vi "Handle Exception.vi"(7 "Processing In":refnum<class "Processing.lvclass">, 8 "error in (no error)":errorcluster, 11 "Authentication Handler in":refnum<class "Authentication Handler.lvclass">) -> (0 "error out":errorcluster, 5 "Processing":refnum<class "Processing.lvclass">)   [LabVIEW 2020, in "HTTP Server.lvlib" / "Authentication Handler.lvclass"]
uses:
  Authentication Handler.lvclass
  Processing/Processing.lvclass
  User/User.lvclass
  C:/dev/lv20CE/relink/lv-http-server/HTTP Server/Service/Service.lvclass
  Processing/Processing.lvclass/Processing.ctl
  Authentication Provider/Authentication Provider.lvclass
  lv-http-util/HTTP Utils/Redirect Response/Redirect Response.lvclass
  C:/dev/lv20CE/relink/lv-http-util/HTTP Utils/Response/Response.lvclass
  Authentication Handler.lvclass/Authentication Handler.ctl
  lv-http-util/HTTP Utils/Response/Response.lvclass
  lv-http-util/HTTP Utils/Request/Request.lvclass
  Session/Session.lvclass
  Values/Values.lvclass
  lv-uri/URI/URI/URI.lvclass
  C:/dev/lv20CE/relink/lv-http-server/HTTP Server/User/User.lvclass
  C:/dev/lv20CE/relink/lv-http-server/HTTP Server/Authentication Provider/Authentication Provider.lvclass
  C:/dev/lv20CE/relink/lv-http-util/HTTP Utils/Redirect Response/Redirect Response.lvclass
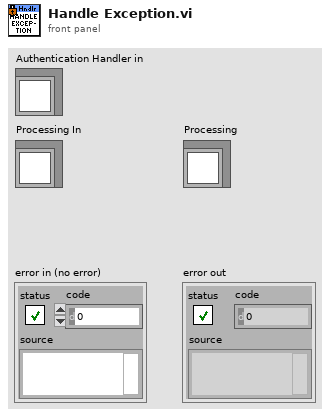
[diagram p1: front panel]
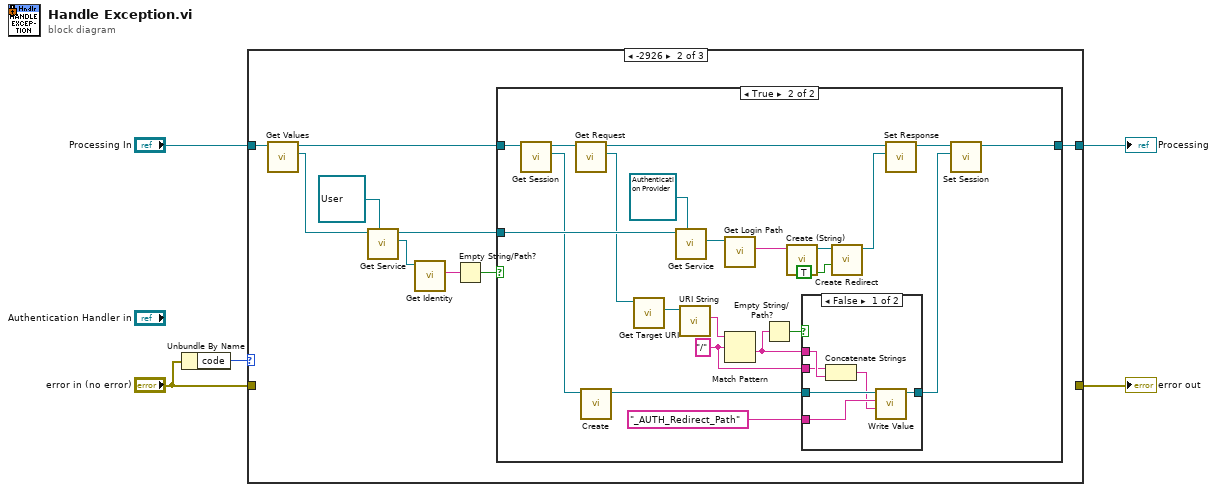
[diagram p0: block diagram]
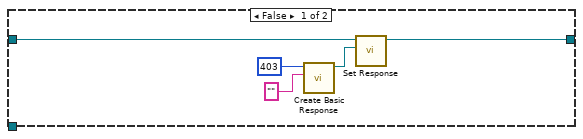
[diagram p3: hidden frame]
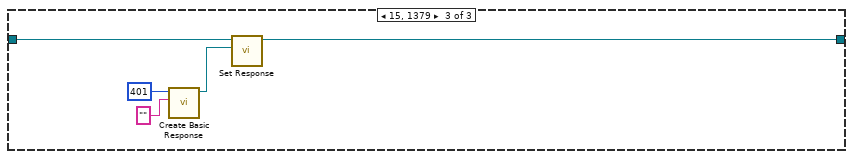
[diagram p5: hidden frame]
diagram:
  n1 = Unbundle By Name("error in (no error)") -> ("code"=w5:i32)
  n2 = case shown="-2926" w5 {
    tunnel: "error in (no error)" -> [w7 _ _]
    tunnel: [w7 _ _] -> w3
    tunnel: "Processing In" -> [w6 w10 w53]
    tunnel: [w6 w11 w51] -> w1
    frame Default {
    }
    frame -2926 {
      n3 = call "Get Values.vi"("Processing in"=w10) -> ("Values"=w9:refnum<class "Values.lvclass">, "Processing out"=w8:refnum<class "Processing.lvclass">)  [unwired: 9 in]
      n4 = call "Get Service.vi"("Service Type"=refnum<class "User.lvclass"> refnum ("HTTP Server.lvlib:User.lvclass"), "Values in"=w9) -> ("Service"=w15:refnum<class "User.lvclass">, "Values out"=w12:refnum<class "Values.lvclass">)  [unwired: 7 in, 1 out]
      n5 = call-dynamic "Get Identity.vi"("User in"=w15) -> ("Identity"=w14:string)  [unwired: 8 in, 2 out]
      n6 = Empty String/Path?(string/path=w14) -> (empty?=w13:bool)
      n7 = case shown="True" w13 {
        tunnel: w12 -> [_ w43]
        tunnel: [w18 w29] -> w11
        tunnel: w8 -> [w17 w25]
        frame False {
          n8 = call "Create Basic Response.vi"("Payload"="", "Status Code"=u16 403) -> ("Response out"=w19:refnum<class "Response.lvclass">)  [unwired: 8 in, 1 out]
          n9 = call "Set Response.vi"("Response"=w19, "Processing in"=w17) -> ("Processing out"=w18:refnum<class "Processing.lvclass">)  [unwired: 9 in]
        }
        frame True {
          w34 = "/" ("regular expression")
          n10 = call "Get Session.vi"("Processing in"=w25) -> ("Session"=w26:refnum<class "Session.lvclass">, "Processing out"=w27:refnum<class "Processing.lvclass">)  [unwired: 9 in]
          n11 = call "Get Request.vi"("Processing in"=w27) -> ("Request"=w33:refnum<class "Request.lvclass">, "Processing out"=w32:refnum<class "Processing.lvclass">)  [unwired: 9 in]
          n12 = call "Create.vi"("Session in"=w26) -> ("Session out"=w28:refnum<class "Session.lvclass">)  [unwired: 9 in, 1 out]
          n13 = call "Get Target URI.vi"("Request in"=w33) -> ("Target URI"=w39:refnum<class "URI.lvclass">)  [unwired: 8 in, 2 out]
          n14 = call "Get Service.vi"("Service Type"=refnum<class "Authentication Provider.lvclass"> refnum ("HTTP Server.lvlib:Authentication Provider.lvclass"), "Values in"=w43) -> ("Service"=w41:refnum<class "Authentication Provider.lvclass">)  [unwired: 7 in, 2 out]
          n15 = call "URI String.vi"("URI in"=w39) -> ("URI String"=w38:string)  [unwired: 9 in, 1 out]
          n16 = call-dynamic "Get Login Path.vi"("Authentication Provider in"=w41) -> ("Login Path"=w40:string)  [unwired: 8 in, 2 out]
          n17 = Match Pattern(string=w38, regular expression=w34) -> (after substring=w37:string)  [unwired: 1 in, 3 out]
          n18 = Empty String/Path?(string/path=w37) -> (empty?=w36:bool)
          n19 = call "Create (String).vi"("URI String"=w40) -> ("URI out"=w24:refnum<class "URI.lvclass">)  [unwired: 9 in, 1 out]
          n20 = case shown="False" w36 {
            tunnel: w37 -> [w46 _]
            tunnel: w28 -> [w49 w50]
            tunnel: "_AUTH_Redirect_Path" ("Name") -> [w48 _]
            tunnel: [w47 w50] -> w30
            tunnel: w34 -> [w45 _]
            frame False {
              n21 = Concatenate Strings(w45, w46) -> (w44:string)
              n22 = call "Write Value.vi"("Value"=w44, "Name"=w48, "Session in"=w49) -> ("Session out"=w47:refnum<class "Session.lvclass">)  [unwired: 6 in, 2 out]
            }
            frame True {
            }
          }
          n23 = call "Create Redirect.vi"("Force GET? (F)"=TRUE, "Redirect URI"=w24) -> ("Redirect Response out"=w22:refnum<class "Redirect Response.lvclass">)  [unwired: 8 in, 1 out]
          n24 = call "Set Response.vi"("Response"=w22, "Processing in"=w32) -> ("Processing out"=w31:refnum<class "Processing.lvclass">)  [unwired: 9 in]
          n25 = call "Set Session.vi"("Session"=w30, "Processing in"=w31) -> ("Processing out"=w29:refnum<class "Processing.lvclass">)  [unwired: 9 in]
        }
      }
    }
    frame 15, 1379 {
      n26 = call "Create Basic Response.vi"("Payload"="", "Status Code"=u16 401) -> ("Response out"=w52:refnum<class "Response.lvclass">)  [unwired: 8 in, 1 out]
      n27 = call "Set Response.vi"("Response"=w52, "Processing in"=w53) -> ("Processing out"=w51:refnum<class "Processing.lvclass">)  [unwired: 9 in]
    }
  }
  "error out" <- w3
  "Processing" <- w1
